vi "UpdateProjectFiles.vi"() -> ()   [LabVIEW 2020, in "veristand-steps-build-tools.lvlib"]
uses:
  veristand-steps-build-tools.lvlib
  <vilib>/Wiresmith Technology/LabVIEW CLI/CLI Class/CLI.lvclass
panel:
  out "error out":errorcluster
  # "This VI is used to build the VeriStand Step Types manually or using an automated build system.\n\nThis VI performs the following actions:\n\n1. Reads the VeriStand Step Types version from the version file in the top level of the repository.\n\n2. Forms staging paths and creates new directories on disk if needed.\n\n3. Updates VeristandSteps.csproj file XML to use correct VeriStand and TestStand .NET assemblies\n\n4. Builds the VeriStandSteps.dll assembly using MSBuild\n\n5. Updates NI_VeristandTypes.ini file XML to new Step Types version\n\n6. Places all built files in appropriate staging directories from step (2)\n\n7. Places documentaion/tutorial files to staging directories created in step (2)."
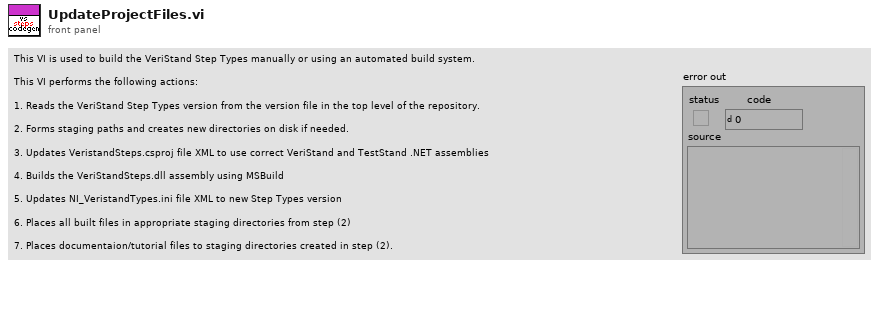
[diagram p1: front panel]
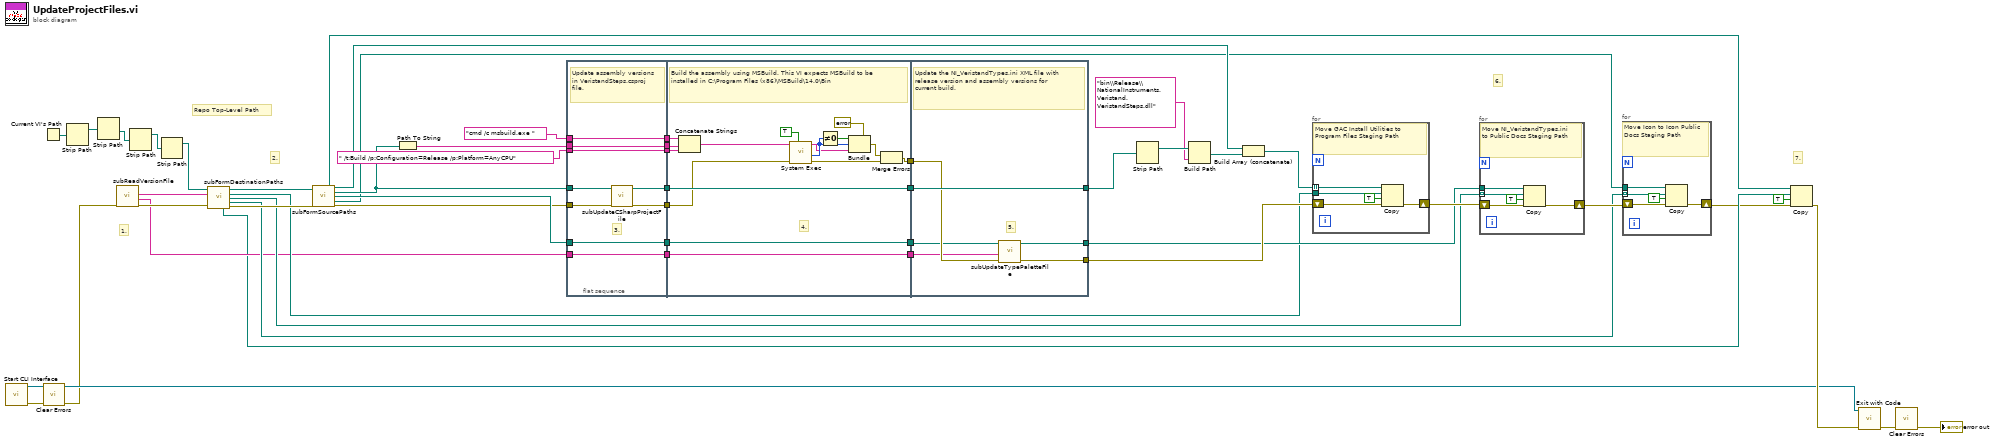
[diagram p0: block diagram]
diagram:
  # "7."
  # "Repo Top-Level Path"
  # "6."
  # "2."
  # "1."
  n1 = call <vilib>:"Start CLI Interface.vi"() -> ("error out"=w4:errorcluster, "CLI out"=w5:refnum<class "CLI.lvclass">)  [unwired: 9 in, 1 out]
  n2 = Current VI's Path() -> (path=w16:path)
  n3 = call <vilib>:"Clear Errors.vi"("error in (no error)"=w4) -> ("error out"=w3:errorcluster)  [unwired: 5 in, 1 out]
  n4 = Strip Path(path=w16) -> (stripped path=w17:path)  [unwired: 1 out]
  n5 = Strip Path(path=w17) -> (stripped path=w18:path)  [unwired: 1 out]
  n6 = call "subReadVersionFile.vi"("error in"=w3) -> ("error out"=w20:errorcluster, "Step Types Version"=w13:string, "TestStand Versions"=w12:string)  [unwired: 8 in]
  n7 = Strip Path(path=w18) -> (stripped path=w19:path)  [unwired: 1 out]
  n8 = Strip Path(path=w19) -> (stripped path=w15:path)  [unwired: 1 out]
  n9 = call "subFormDestinationPaths.vi"("Repo Top-Level Path"=w15, "TestStand Version String"=w12, "error in"=w20) -> ("Repo Top-Level Path out"=w14:path, "Program Files Destination Path"=w23:path, "TypePalettes Paths"=w21:path[], "Icon Paths"=w22:path[], "VS Steps Pub Docs Path"=w9:path, "error out"=w24:errorcluster)  [unwired: 7 in]
  n10 = call "subFormSourcePaths.vi"("Repo Top-level"=w14, "error in (no error)"=w24) -> ("Documentation Source Path"=w10:path, "GACUtilityPaths"=w28:path[], "CSharp Assembly Project Path"=w27:path, "TypePalette File Path"=w26:path, "Icon File Path"=w11:path, "error out"=w25:errorcluster)  [unwired: 8 in]
  n11 = Path To String(path=w27) -> (string=w36:string)
  n12 = flat-sequence {
    tunnel: " /t:Build /p:Configuration=Release /p:Platform=AnyCPU" ("string") -> [w59]
    tunnel: "cmd /c msbuild.exe " -> [w60]
    tunnel: [w60] -> w48
    tunnel: [w59] -> w47
    tunnel: w27 -> [w58]
    tunnel: [w57] -> w46
    tunnel: [w56] -> w45
    tunnel: w36 -> [w55]
    tunnel: [w55] -> w35
    tunnel: w26 -> [w54]
    tunnel: [w54] -> w33
    tunnel: w13 -> [w53]
    tunnel: [w53] -> w32
    tunnel: w25 -> [w52]
    tunnel: [w76] -> w43
    tunnel: w45 -> [w76]
    tunnel: w46 -> [w71]
    tunnel: w47 -> [w73]
    tunnel: w48 -> [w74]
    tunnel: [w62] -> w42
    tunnel: w35 -> [w70]
    tunnel: [w69] -> w34
    tunnel: w33 -> [w69]
    tunnel: w32 -> [w68]
    tunnel: [w68] -> w31
    tunnel: [w82] -> w29
    tunnel: w43 -> [w82]
    tunnel: [w81] -> w41
    tunnel: w42 -> [w80]
    tunnel: w34 -> [w78]
    tunnel: w31 -> [w79]
    tunnel: [w77] -> w30
    frame #0 {
      # "3."
      # "Update assembly versions in VeristandSteps.csproj file."
      n13 = call "subUpdateCSharpProjectFile.vi"("error in (no error)"=w52, ".csproj path"=w58) -> ("error out"=w57:errorcluster, ".csproj path out"=w56:path)  [unwired: 8 in]
    }
    frame #1 {
      # "4."
      # "Build the assembly using MSBuild. This VI expects MSBuild to be installed in C:\\Program Files (x86)\\MSBuild\\14.0\\Bin"
      n14 = Concatenate Strings(w74, w70, w73) -> (w72:string)
      n15 = call <vilib>:"System Exec.vi"("wait until completion? (T)"=TRUE, "error in (no error)"=w71, "command line"=w72) -> ("error out"=w63:errorcluster, "return code"=w66:i32, "standard output"=w61:string)  [unwired: 5 in, 1 out]
      n16 = Not Equal To 0?(x=w66) -> (x != 0?=w65:bool)
      n17 = Bundle(cluster=errorcluster {"status"=FALSE, "code"=0, "source"=""} ("error constant"), "status"=w65, "code"=w66, "source"=w61) -> (w64:errorcluster)
      n18 = Merge Errors(w64, w63) -> (w62:errorcluster)
    }
    frame #2 {
      # "5."
      # "Update the NI_VeristandTypes.ini XML file with release version and assembly versions for current build."
      n19 = call "subUpdateTypePaletteFile.vi"("error in (no error)"=w80, "Step Types Version"=w79, "TypePalette .ini file location"=w78) -> ("error out"=w81:errorcluster, "Type Palettes File Path out"=w77:path)  [unwired: 7 in]
    }
  }
  n20 = Strip Path(path=w29) -> (stripped path=w50:path)  [unwired: 1 out]
  n21 = Build Path(base path=w50, name or relative path="bin\\Release\\NationalInstruments.Veristand.VeristandSteps.dll") -> (appended path=w40:path)
  n22 = Build Array (concatenate)(w28, w40) -> (w39:path[])
  n23 = for {
    shift-right: [w87] -> w38
    shift-left: w41 -> [w86]
    tunnel: w39 -> [w85] mode=indexing
    tunnel: w23 -> [w84]
    # "Move GAC Install Utilities to Program Files Staging Path"
    n24 = Copy(8:w86, 9:TRUE ("overwrite (F)"), 10:w84, 11:w85) -> (0:w87:errorcluster)  [unwired: 1 in, 2 out]
  }
  n25 = for {
    shift-right: [w92] -> w37
    shift-left: w38 -> [w91]
    tunnel: w30 -> [w89]
    tunnel: w21 -> [w88] mode=indexing
    # "Move NI_VeristandTypes.ini to Public Docs Staging Path"
    n26 = Copy(8:w91, 9:TRUE ("overwrite (F)"), 10:w88, 11:w89) -> (0:w92:errorcluster)  [unwired: 1 in, 2 out]
  }
  n27 = for {
    shift-right: [w97] -> w8
    shift-left: w37 -> [w96]
    tunnel: w22 -> [w94] mode=indexing
    tunnel: w11 -> [w93]
    # "Move Icon to Icon Public Docs Staging Path"
    n28 = Copy(8:w96, 9:TRUE ("overwrite (F)"), 10:w94, 11:w93) -> (0:w97:errorcluster)  [unwired: 1 in, 2 out]
  }
  n29 = Copy(8:w8, 9:TRUE ("overwrite (F)"), 10:w9, 11:w10) -> (0:w6:errorcluster)  [unwired: 1 in, 2 out]
  n30 = call <vilib>:"Exit with Code.vi"("error in (no error)"=w6, "CLI in"=w5) -> ("error out"=w2:errorcluster)  [unwired: 9 in]
  n31 = call <vilib>:"Clear Errors.vi"("error in (no error)"=w2) -> ("error out"=→"error out":errorcluster)  [unwired: 5 in, 1 out]
